vi "Main.vi"() -> ()   [LabVIEW 2017]
doc: "Use this template to build a simple state machine design pattern. Each state executes code and determines which state to transition to."
uses:
  controls/State.ctl
  controls/Data.ctl
  <vilib>/measure/mascope.llb/Amplitude and Levels 1 chan.vi
  <vilib>/Analysis/NI_AALBase.lvlib
  <vilib>/measure/NI_MAPro.lvlib
panel:
  out "High state level measured":dbl
  out "Amplitude measured":dbl
  in  "state setting":T1
  out "Waveform Graph":dbl[](graph)
  in  "Amplitude":dbl
  in  "Analyze Data":bool
  in  "Accquire Data":bool
  in  "Exit":bool
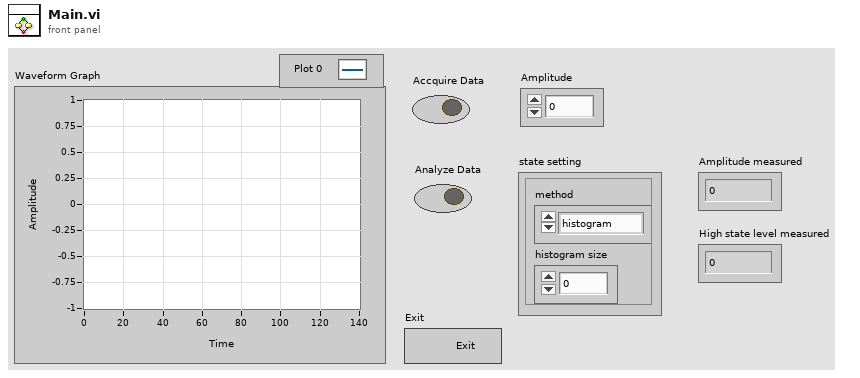
[diagram p1: front panel]
types:
  T1 = cluster{"histogram size":dbl, "method":enum16{"histogram", "peak", "auto select"}, "histogram method":enum16{"mode"}, "reserved":dbl}
  T2 = typedef "Data.ctl" = cluster{"Boolean <Replace Me>":bool, "String <Replace Me>":string, "Numeric <Replace Me>":dbl}
  T3 = typedef "State.ctl" = enum16{"Initialize", "Wait for Event", "Acquire Data", "Analyze Data", "Exit"}
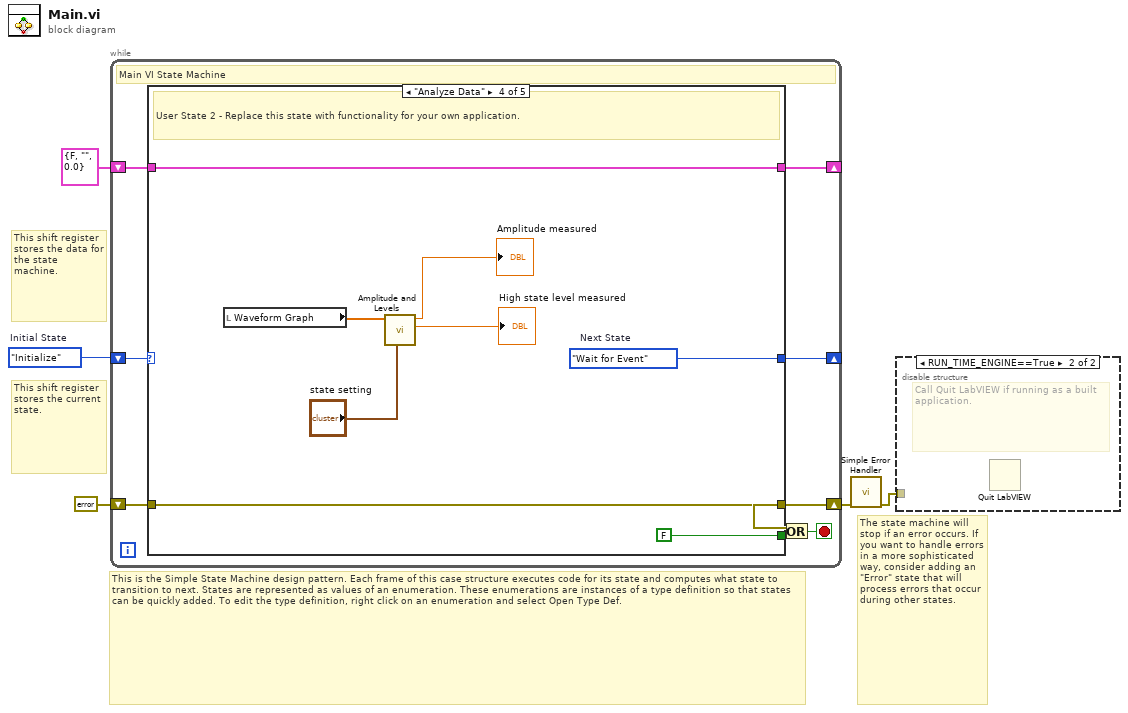
[diagram p0: block diagram]
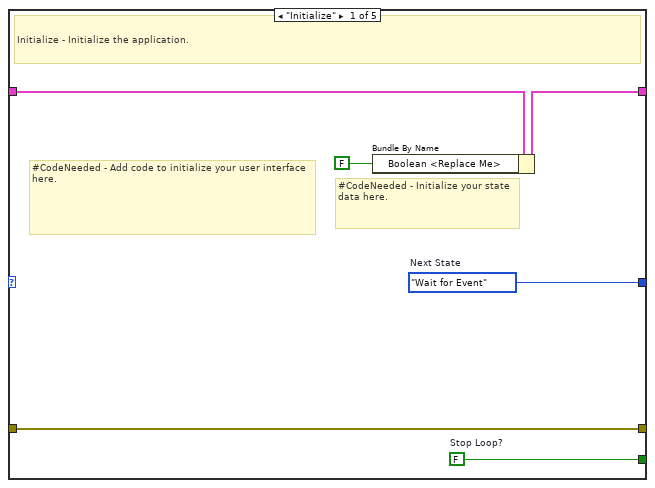
[diagram p3: hidden frame]
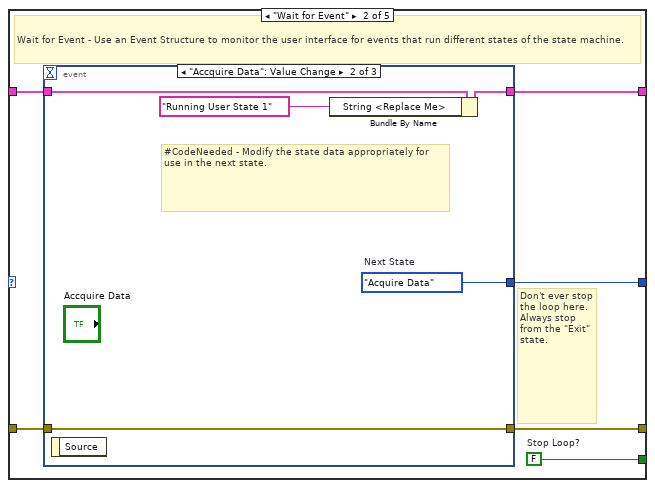
[diagram p4: hidden frame]
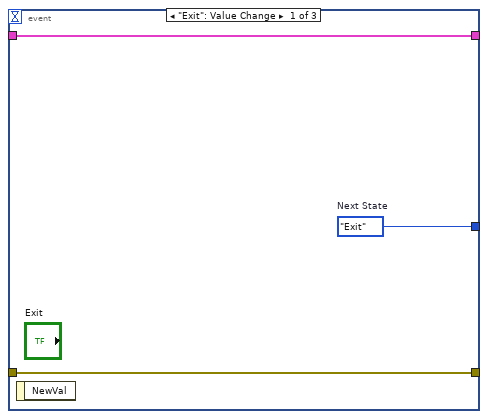
[diagram p5: hidden frame]
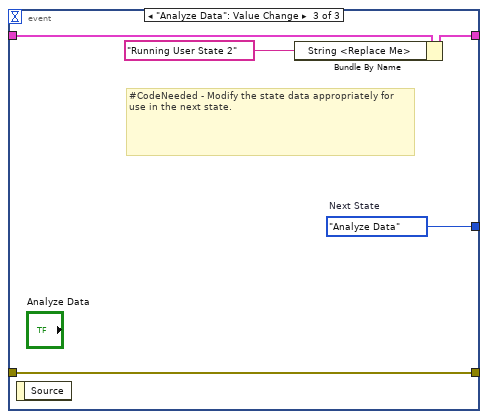
[diagram p6: hidden frame]
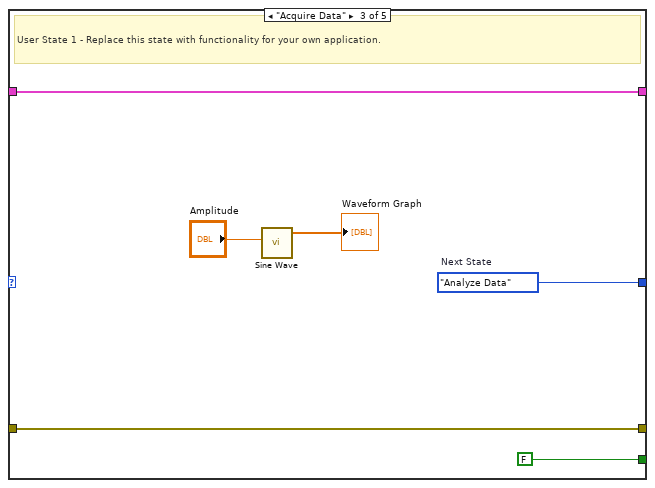
[diagram p7: hidden frame]
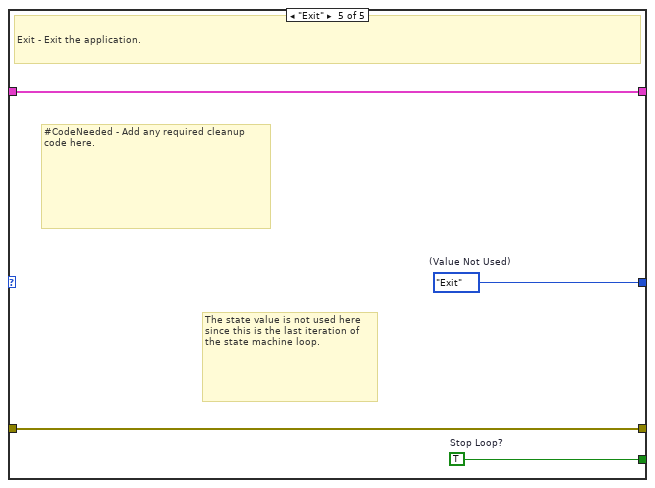
[diagram p8: hidden frame]
diagram:
  w5 = State."Initialize"  # Initial State
  # "The state machine will stop if an error occurs. If you want to handle errors in a more sophisticated way, consider adding an \"Error\" state that will process errors that occur during other states."
  # "This shift register stores the data for the state machine."
  # "This is the Simple State Machine design pattern. Each frame of this case structure executes code for its state and computes what state to transition to next. States are represented as values of an enumeration. These enumerations are instances of a type definition so that states can be quickly added. To edit the type definition, right click on an enumeration and select Open Type Def."
  # "This shift register stores the current state."
  n1 = while {
    shift-right: [w12] -> _
    shift-left: w5 -> [w13]
    shift-right: [w10] -> _
    shift-left: T2 {"Boolean <Replace Me>"=FALSE, "String <Replace Me>"="", "Numeric <Replace Me>"=0.0} ("Data") -> [w11]
    shift-right: [w6] -> w2
    shift-left: errorcluster {"status"=FALSE, "code"=0, "source"=""} ("error constant") -> [w9]
    stop <- w7 stop-if-true
    # "Main VI State Machine"
    n2 = case shown="\"Analyze Data\"" w13 {
      tunnel: [w19 w25 w44 w52 w56] -> w12
      tunnel: [w18 w24 FALSE ("Stop Loop?") FALSE ("Stop Loop?") w54] -> w8
      tunnel: w11 -> [w17 w23 w42 w50 w55]
      tunnel: [w16 w22 w42 w50 w55] -> w10
      tunnel: w9 -> [w14 w21 w41 w49 w53]
      tunnel: [w14 w20 w41 w49 w53] -> w6
      frame "Initialize" {
        w18 = FALSE  # Stop Loop?
        w19 = State."Wait for Event"  # Next State
        # "#CodeNeeded - Initialize your state data here."
        # "#CodeNeeded - Add code to initialize your user interface here."
        # "Initialize - Initialize the application."
        n3 = Bundle By Name(cluster=w17, "Boolean <Replace Me>"=FALSE ("Replace_Me_Boolean")) -> (w16:T2)
      }
      frame "Wait for Event" {
        w24 = FALSE  # Stop Loop?
        # "Don't ever stop the loop here. Always stop from the \"Exit\" state."
        # "Wait for Event - Use an Event Structure to monitor the user interface for events that run different states of the state machine."
        n4 = event shown="[1] \"Accquire Data\": Value Change" {
          selector: _ -> [_ _ _]
          dyn-events: _ -> [_ _ _]
          timeout: _ -> [_ _ _]
          tunnel: [w28 w33 w38] -> w25
          tunnel: w23 -> [w27 w32 w37]
          tunnel: [w27 w31 w36] -> w22
          tunnel: w21 -> [w26 w29 w34]
          tunnel: [w26 w29 w34] -> w20
          event "Exit": Value Change {
            w28 = State."Exit"  # Next State
            n5 = event-data() -> ()  [unwired: 1 in, 1 out]
          }
          event "Accquire Data": Value Change {
            w33 = State."Acquire Data"  # Next State
            # "#CodeNeeded - Modify the state data appropriately for use in the next state."
            n6 = event-data() -> ()  [unwired: 1 in, 1 out]
            n7 = Bundle By Name(cluster=w32, "String <Replace Me>"="Running User State 1" ("Running User State 1")) -> (w31:T2)
          }
          event "Analyze Data": Value Change {
            w38 = State."Analyze Data"  # Next State
            # "#CodeNeeded - Modify the state data appropriately for use in the next state."
            n8 = event-data() -> ()  [unwired: 1 in, 1 out]
            n9 = Bundle By Name(cluster=w37, "String <Replace Me>"="Running User State 2" ("Running User State 2")) -> (w36:T2)
          }
        }
      }
      frame "Acquire Data" {
        w44 = State."Analyze Data"  # Next State
        # "User State 1 - Replace this state with functionality for your own application."
        n10 = call <vilib>:"Sine Wave.vi"("amplitude"="Amplitude") -> ("sine wave"=→"Waveform Graph":dbl[])  [unwired: 4 in, 2 out]
      }
      frame "Analyze Data" {
        w52 = State."Wait for Event"  # Next State
        # "User State 2 - Replace this state with functionality for your own application."
        n11 = local read "Waveform Graph"() -> (w48:dbl[])
        n12 = call-poly <vilib>:"Amplitude and Levels.vi"("state settings"="state setting", "signal in"=w48) -> ("high state level"=→"High state level measured":dbl, "amplitude"=→"Amplitude measured":dbl)  [unwired: 6 in, 2 out]
      }
      frame "Exit" {
        w54 = TRUE  # Stop Loop?
        w56 = State."Exit"  # (Value Not Used)
        # "#CodeNeeded - Add any required cleanup code here."
        # "The state value is not used here since this is the last iteration of the state machine loop."
        # "Exit - Exit the application."
      }
    }
    n13 = Or(x=w6, y=w8) -> (x .or. y?=w7:bool)
  }
  n14 = call <vilib>:"Simple Error Handler.vi"("error in (no error)"=w2) -> ("error out"=w1:errorcluster)  [unwired: 4 in, 4 out]
  n15 = disable-structure shown="RUN_TIME_ENGINE==True" {
    disable-tunnel: w1 -> [_ _]
    frame condition #0 (active) {
    }
    frame condition #1 {
      # "Call Quit LabVIEW if running as a built application."
      n16 = Quit LabVIEW() -> ()  [unwired: 1 in]
    }
  }
